vi "Facade.vi"(0 "Data In":T4, 2 "Display State In":T2, 3 "Container State":T3) -> (6 "Data Out":T4, 7 "Display State Out":T2, 8 "Action":T1)   [LabVIEW 2017, in "XTriPhaseGraph.xctl"]
uses:
  XTriPhaseGraph.xctl
  Data.ctl
  <vilib>/_xctls/Container State.ctl
  State.ctl
  <vilib>/_xctls/Action.ctl
  <vilib>/Utility/miscctls.llb/LVForegroundBackgroundColorsTypeDef.ctl
  <vilib>/_xctls/XControlSupport.lvlib
panel:
  out "wf A":waveform(dbl)(graph)
  out "wf B":waveform(dbl)(graph)
  out "wf C":waveform(dbl)(graph)
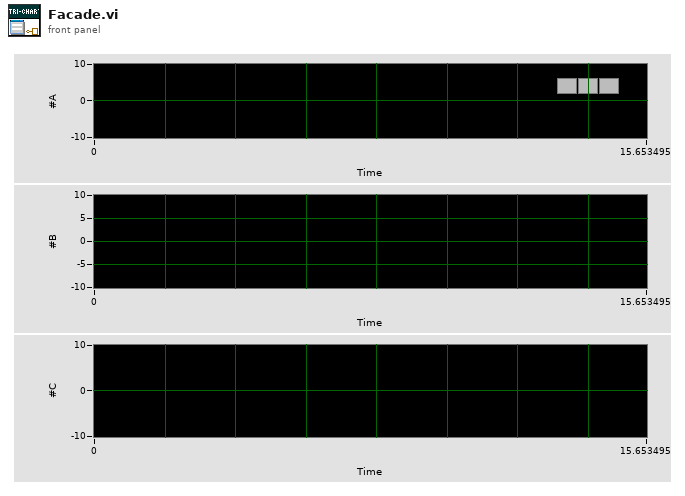
[diagram p1: front panel]
types:
  T1 = typedef "XControlSupport.lvlib/Action.ctl" = cluster{"Data Changed?":bool, "State Changed?":bool, "Action Name":string}
  T2 = typedef "XTriPhaseGraph.xctl/State.ctl" = cluster{"Labels":string[], "X Label":string}
  T3 = typedef "XControlSupport.lvlib/Container State.ctl" = cluster{"Indicator?":bool, "Run Mode?":bool, " Refnum":refnum<vi>}
  T4 = typedef "XTriPhaseGraph.xctl/Data.ctl" = waveform(dbl)[]
  T5 = cluster{"wf A":refnum<vi>, "wf B":refnum<vi>, "wf C":refnum<vi>, "Splitter":refnum<vi>, "Splitter 2":refnum<vi>}
  T6 = typedef "LVRectTypeDef.ctl" = cluster{"Left":i16, "Top":i16, "Right":i16, "Bottom":i16}
  T7 = typedef "LVRangeTypeDef.ctl" = cluster{"Minimum":dbl, "Maximum":dbl, "Increment":dbl, "Minor Increment":dbl, "Start":dbl}
  T8 = typedef "LVForegroundBackgroundColorsTypeDef.ctl" = cluster{"Foreground Color":u32, "Background Color":u32}
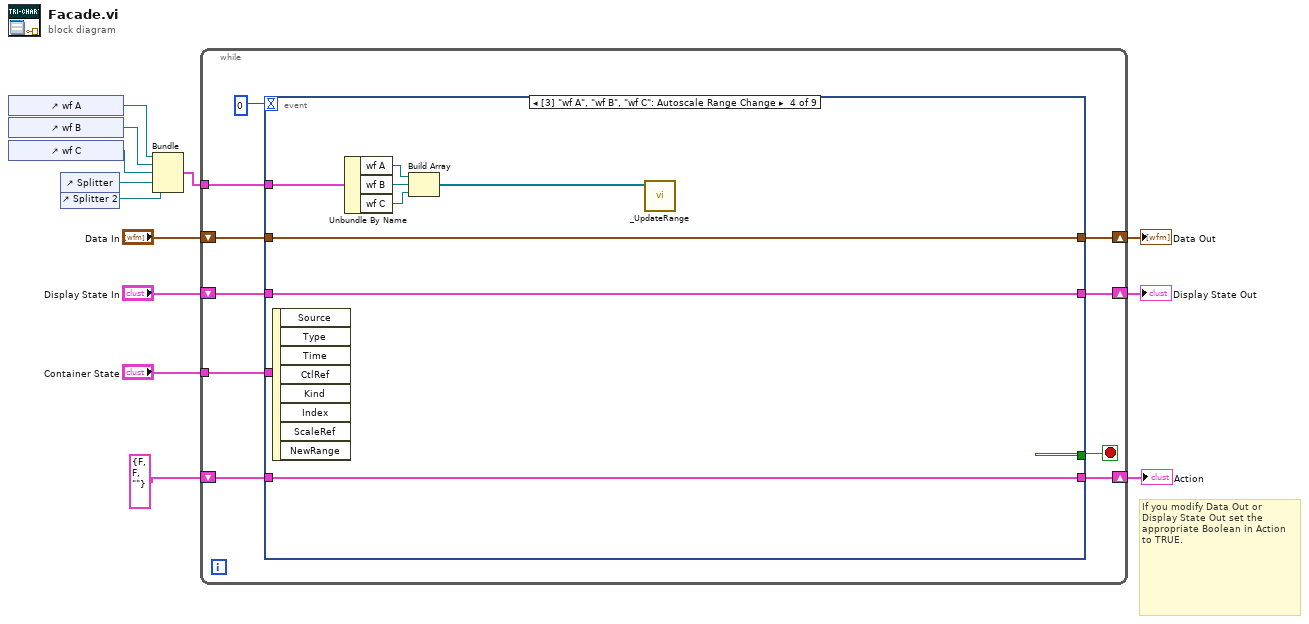
[diagram p0: block diagram]
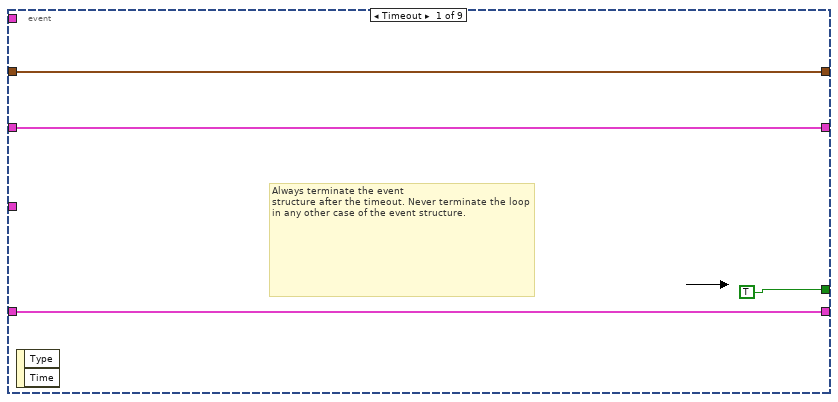
[diagram p2: hidden frame]
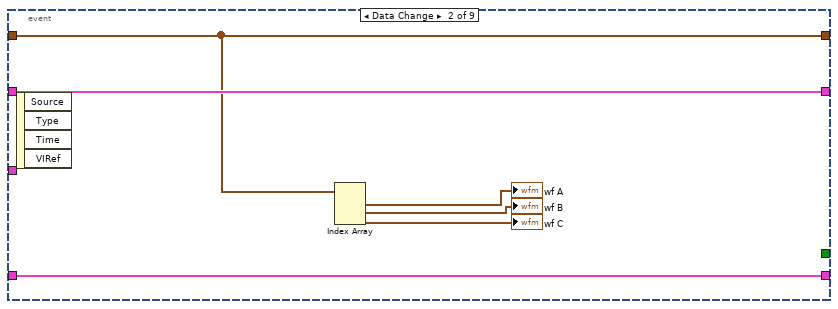
[diagram p3: hidden frame]
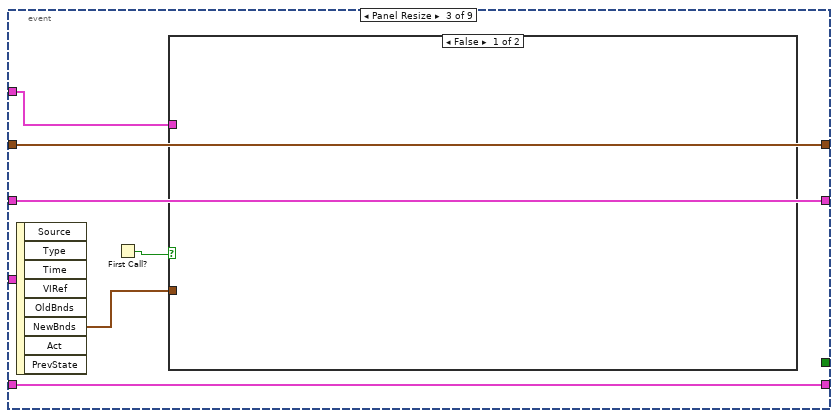
[diagram p4: hidden frame]
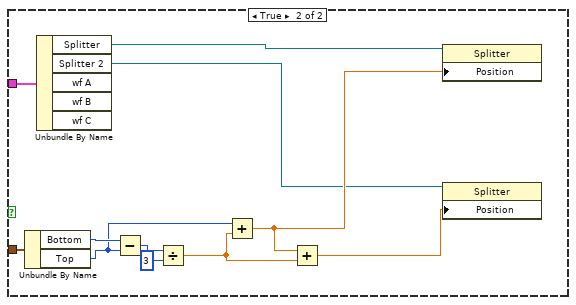
[diagram p5: hidden frame]
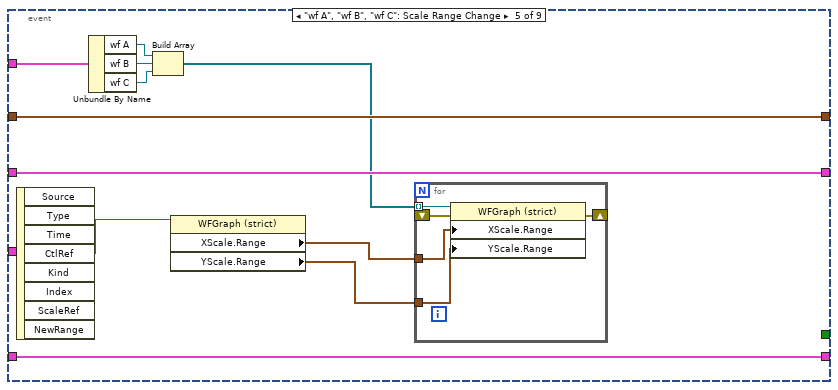
[diagram p6: hidden frame]
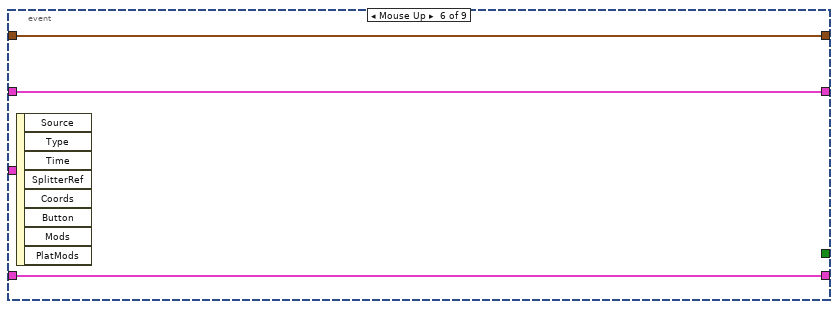
[diagram p7: hidden frame]
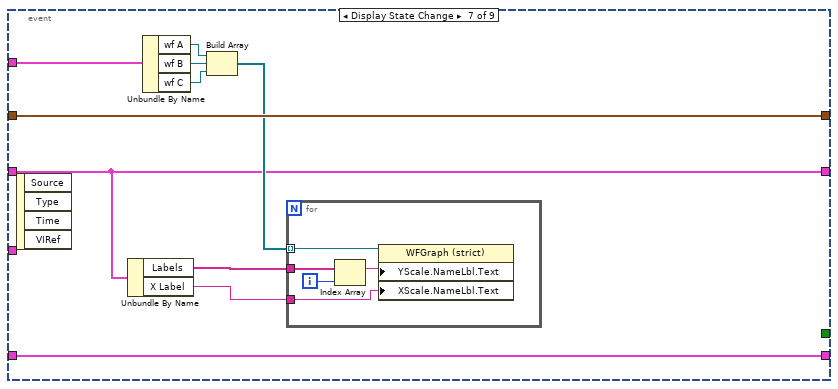
[diagram p8: hidden frame]
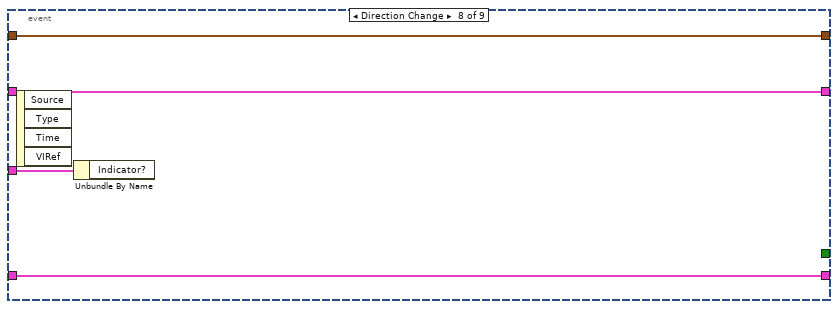
[diagram p9: hidden frame]
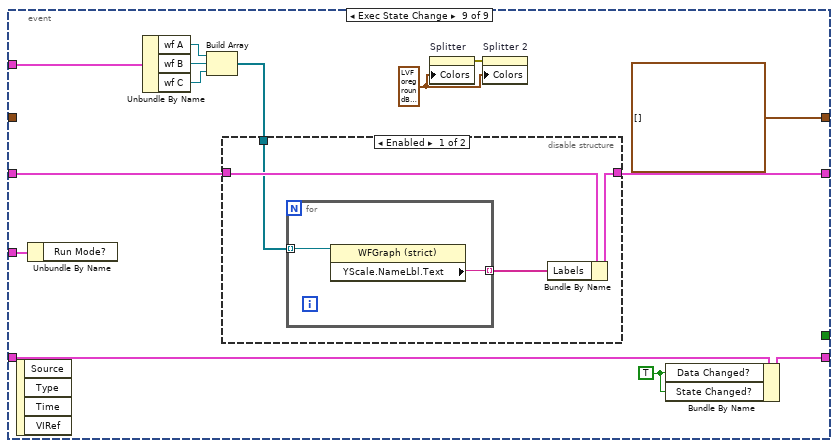
[diagram p10: hidden frame]
diagram:
  # "If you modify Data Out or\nDisplay State Out set the\nappropriate Boolean in Action\nto TRUE."
  n1 = control-ref of="wf A"() -> (w3:refnum<vi>)
  n2 = control-ref of="wf B"() -> (w2:refnum<vi>)
  n3 = control-ref of="wf C"() -> (w1:refnum<vi>)
  n4 = control-ref of="Splitter"() -> (w6:refnum<vi>)
  n5 = control-ref of="Splitter 2"() -> (w5:refnum<vi>)
  n6 = Bundle("wf A"=w3, "wf B"=w2, "wf C"=w1, "Splitter"=w6, "Splitter 2"=w5) -> (w4:T5)  [unwired: 1 in]
  n7 = while {
    shift-right: [w22] -> w10
    shift-left: "Display State In" -> [w23]
    tunnel: "Container State" -> [w19]
    shift-right: [w17] -> w13
    shift-left: "Data In" -> [w18]
    shift-right: [w15] -> w8
    shift-left: T1 {"Data Changed?"=FALSE, "State Changed?"=FALSE, "Action Name"=""} ("Action") -> [w16]
    tunnel: w4 -> [w14]
    stop <- w21 stop-if-true
    n8 = event shown="[3] \"wf A\", \"wf B\", \"wf C\": Autoscale Range Change" {
      selector: _ -> [_ _ _ _ _ _ _ _ _]
      dyn-events: _ -> [_ _ _ _ _ _ _ _ _]
      timeout: 0 -> [_ _ _ _ _ _ _ _ _]
      tunnel: w23 -> [w25 w33 w39 w58 w69 w77 w80 w95 w109]
      tunnel: [w25 w33 w39 w58 w69 w77 w80 w95 w99] -> w22
      tunnel: [TRUE _ _ _ _ _ _ _ _] -> w21
      tunnel: w19 -> [_ _ _ _ _ _ _ w96 w110]
      tunnel: w18 -> [w24 w28 w38 w57 w68 w76 w86 w94 _]
      tunnel: [w24 w28 w38 w57 w68 w76 w86 w94 T4 [] ("Data In")] -> w17
      tunnel: [w26 w32 w37 w56 w67 w75 w87 w93 w106] -> w15
      tunnel: w16 -> [w26 w32 w37 w56 w67 w75 w87 w93 w108]
      tunnel: w14 -> [_ _ w35 w55 w66 _ w81 _ w101]
      event Timeout {
        # "Always terminate the event\nstructure after the timeout. Never terminate the loop in any other case of the event structure."
        n9 = event-data() -> ()  [unwired: 1 in, 2 out]
      }
      event Data Change {
        n10 = event-data() -> ()  [unwired: 1 in, 4 out]
        n11 = Index Array(array=w28) -> (element #1=→"wf A":waveform(dbl), element #2=→"wf B":waveform(dbl), element #3=→"wf C":waveform(dbl))  [unwired: 3 in]
      }
      event Panel Resize {
        n12 = event-data() -> ("NewBnds"=w36:T6)  [unwired: 1 in, 7 out]
        n13 = First Call?() -> (First Call?: T/F=w34:bool)
        n14 = case shown="False" w34 {
          tunnel: w36 -> [_ w50]
          tunnel: w35 -> [_ w45]
          frame False {
          }
          frame True {
            n15 = Unbundle By Name(w50) -> ("Bottom"=w47:i16, "Top"=w40:i16)
            n16 = Unbundle By Name(w45) -> ("Splitter"=w41:refnum<vi>, "Splitter 2"=w42:refnum<vi>)  [unwired: 3 out]
            n17 = Subtract(x=w47, y=w40) -> (x-y=w49:i16)
            n18 = Divide(x=w49, y=i16 3) -> (x/y=w46:dbl)
            n19 = Add(x=w40, y=w46) -> (x+y=w44:dbl)
            n20 = Add(x=w44, y=w46) -> (x+y=w43:dbl)
            n21 = property class="Splitter"(reference=w41, "Position"=w44) -> ()  [unwired: 1 in, 2 out]
            n22 = property class="Splitter"(reference=w42, "Position"=w43) -> ()  [unwired: 1 in, 2 out]
          }
        }
      }
      event "wf A", "wf B", "wf C": Autoscale Range Change {
        n23 = event-data() -> ()  [unwired: 1 in, 8 out]
        n24 = Unbundle By Name(w55) -> ("wf A"=w51:refnum<vi>, "wf B"=w54:refnum<vi>, "wf C"=w53:refnum<vi>)
        n25 = Build Array(w51, w54, w53) -> (w52:refnum<vi>[])
        n26 = call "_UpdateRange.vi"("Array"=w52) -> ()  [unwired: 11 in]
      }
      event "wf A", "wf B", "wf C": Scale Range Change {
        n27 = event-data() -> ("CtlRef"=w61:refnum<vi>)  [unwired: 1 in, 7 out]
        n28 = Unbundle By Name(w66) -> ("wf A"=w63:refnum<vi>, "wf B"=w65:refnum<vi>, "wf C"=w64:refnum<vi>)
        n29 = Build Array(w63, w65, w64) -> (w62:refnum<vi>[])
        n30 = property class="WFGraph (strict)"(reference=w61) -> ("XScale.Range"=w60:T7, "YScale.Range"=w59:T7)  [unwired: 1 in, 2 out]
        n31 = for {
          tunnel: w60 -> [w73]
          tunnel: w59 -> [w72]
          tunnel: w62 -> [w71] mode=indexing
          shift-right: [w70] -> _
          shift-left: _ -> [w74]
          n32 = property class="WFGraph (strict)"(reference=w71, error in=w74, "XScale.Range"=w73, "YScale.Range"=w72) -> (error out=w70:errorcluster)  [unwired: 1 out]
        }
      }
      event Mouse Up {
        n33 = event-data() -> ()  [unwired: 1 in, 8 out]
      }
      event Display State Change {
        n34 = event-data() -> ()  [unwired: 1 in, 4 out]
        n35 = Unbundle By Name(w80) -> ("Labels"=w79:string[], "X Label"=w78:string)
        n36 = Unbundle By Name(w81) -> ("wf A"=w83:refnum<vi>, "wf B"=w85:refnum<vi>, "wf C"=w84:refnum<vi>)
        n37 = Build Array(w83, w85, w84) -> (w82:refnum<vi>[])
        n38 = for {
          tunnel: w82 -> [w92] mode=indexing
          tunnel: w79 -> [w91]
          tunnel: w78 -> [w88]
          i -> [w89]
          n39 = Index Array(array=w91, index=w89) -> (element=w90:string)
          n40 = property class="WFGraph (strict)"(reference=w92, "YScale.NameLbl.Text"=w90, "XScale.NameLbl.Text"=w88) -> ()  [unwired: 1 in, 2 out]
        }
      }
      event Direction Change {
        n41 = event-data() -> ()  [unwired: 1 in, 4 out]
        n42 = Unbundle By Name(w96) -> ()  [unwired: 1 out]
      }
      event Exec State Change {
        w97 = T8 {"Foreground Color"=16777216, "Background Color"=16777216} ("Colors")
        w105 = TRUE ("Data Changed?")
        n43 = event-data() -> ()  [unwired: 1 in, 4 out]
        n44 = Unbundle By Name(w110) -> ()  [unwired: 1 out]
        n45 = Unbundle By Name(w101) -> ("wf A"=w102:refnum<vi>, "wf B"=w104:refnum<vi>, "wf C"=w103:refnum<vi>)
        n46 = Build Array(w102, w104, w103) -> (w100:refnum<vi>[])
        n47 = disable-structure shown="Enabled" {
          disable-tunnel: w109 -> [w114 w117]
          disable-tunnel: w100 -> [w113 _]
          disable-tunnel: [w112 w117] -> w99
          frame Enabled {
            n48 = for {
              tunnel: w113 -> [w116] mode=indexing
              tunnel: [w115] -> w111 mode=indexing
              n49 = property class="WFGraph (strict)"(reference=w116) -> ("YScale.NameLbl.Text"=w115:string)  [unwired: 1 in, 2 out]
            }
            n50 = Bundle By Name(cluster=w114, "Labels"=w111) -> (w112:T2)
          }
          frame Disabled {
          }
        }
        n51 = property on="Splitter" class="Splitter"("Colors"=w97) -> (error out=w98:errorcluster)  [unwired: 2 in, 1 out]
        n52 = property on="Splitter 2" class="Splitter"(error in=w98, "Colors"=w97) -> ()  [unwired: 1 in, 2 out]
        n53 = Bundle By Name(cluster=w108, "Data Changed?"=w105, "State Changed?"=w105) -> (w106:T1)
      }
    }
  }
  "Display State Out" <- w10
  "Data Out" <- w13
  "Action" <- w8
